vi "When Write.vi"(0 "error out":errorcluster, 2 "return count":u32, 11 "Serial in":refnum<class "Mock Serial.lvclass">) -> (3 "Serial out":refnum<class "Mock Serial.lvclass">)   [LabVIEW 2020, in "Mock Serial.lvclass"]
uses:
  Mock Serial.lvclass
  Mock Serial.lvclass/Mock Serial.ctl
  C:/git/astemes-lmock/source/Framework/Mock/LMock Mock.lvclass
  C:/git/astemes-lmock/source/Examples/Serial Driver/Mock Serial/Mock Serial.lvclass
  C:/git/astemes-lmock/source/Examples/Serial Driver/Serial/Serial.lvclass/Serial.lvclass
  Framework/Mock/LMock Mock.lvclass
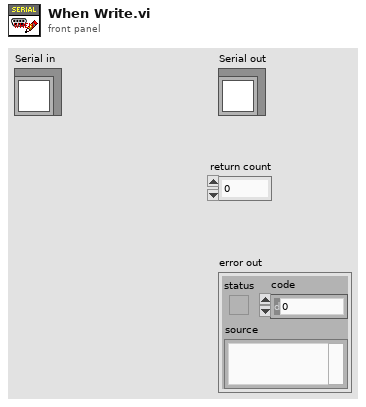
[diagram p1: front panel]
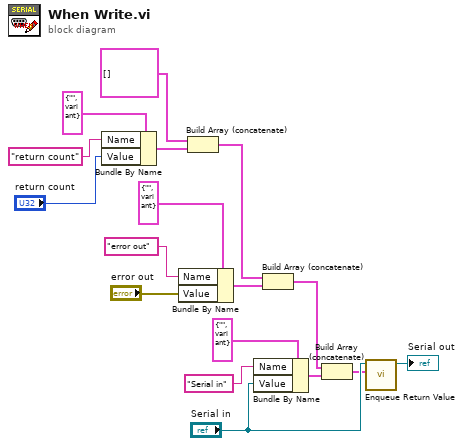
[diagram p0: block diagram]
diagram:
  n1 = Bundle By Name(cluster=cluster{"Name":string, "Value":variant} {"Name"="", "Value"=variant} ("element"), "Name"="return count", "Value"="return count") -> (w5:cluster{"Name":string, "Value":variant})
  n2 = Bundle By Name(cluster=cluster{"Name":string, "Value":variant} {"Name"="", "Value"=variant} ("element"), "Name"="error out", "Value"="error out") -> (w3:cluster{"Name":string, "Value":variant})
  n3 = Build Array (concatenate)(cluster{"Name":string, "Value":variant}[] [] ("Control Values"), w5) -> (w10:cluster{"Name":string, "Value":variant}[])
  n4 = Bundle By Name(cluster=cluster{"Name":string, "Value":variant} {"Name"="", "Value"=variant} ("element"), "Name"="Serial in", "Value"="Serial in") -> (w1:cluster{"Name":string, "Value":variant})
  n5 = Build Array (concatenate)(w10, w3) -> (w13:cluster{"Name":string, "Value":variant}[])
  n6 = Build Array (concatenate)(w13, w1) -> (w15:cluster{"Name":string, "Value":variant}[])
  n7 = call "Enqueue Return Value.vi"("Indicator Values"=w15, "Mock In"="Serial in") -> ("Mock Out"=→"Serial out":refnum<class "Mock Serial.lvclass">)  [unwired: 8 in, 1 out]
